vi "Adjust Splitter.vi"(8 "error in":errorcluster, 10 "Show":bool, 11 "Docking in":refnum<class "Docking.lvclass">) -> (0 "error out":errorcluster, 3 "Docking out":refnum<class "Docking.lvclass">)   [LabVIEW 2023, in "Docking.lvlib" / "Docking.lvclass"]
doc: "This class is designed so that ancestor classes can rescale the UI to fit the actor core of the ancestor UI."
uses:
  Docking.lvclass
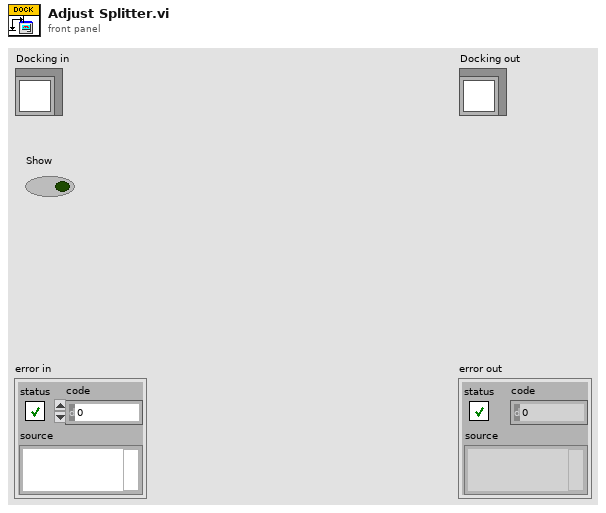
[diagram p1: front panel]
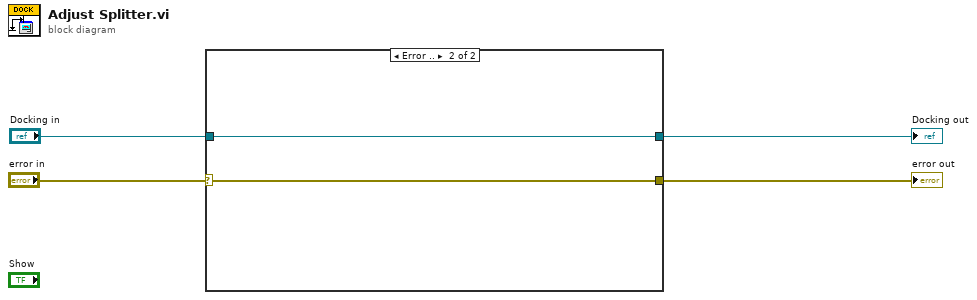
[diagram p0: block diagram]
diagram:
  n1 = case shown="Error .." "error in" {
    selector: "error in" -> [w6 w7]
    tunnel: [w6 w7] -> w3
    tunnel: "Docking in" -> [w5 w8]
    tunnel: [w5 w8] -> w1
    frame No Error {
    }
    frame Error {
    }
  }
  "error out" <- w3
  "Docking out" <- w1
